vi "dfd_Render TF Polynomial.vi"(4 "alignment(left, top)":T2={"horizontal"=enum."left", "vertical"=enum."bottom"}, 5 "format string":string="%.0f", 6 "rendering options":T1, 7 "Fonts Input":T3(array[cluster]), 8 "variable":string="s", 9 "origin":cluster{"x":i16, "y":i16}={"x"=60, "y"=30}, 10 "coefficients":dbl[](array[numeric]) format="%.2f", 11 "picture in":picture) -> (2 "text rect":T4={"left"=60, "top"=13, "right"=157, "bottom"=30}, 3 "rendered equation":picture)   [LabVIEW 2017, in "NI_DigFilter_Process.lvlib"]
doc: "This VI allow to render Polynomials in Picture Control in ascending/descending order of coefficients, ascending/descending order of polynomial and with negative coefficients."
uses:
  <vilib>/addons/Digital Filter Design/NI_DigFilter_Process.lvlib
panel:
  in  "Fonts Defaut":T3(array[cluster])=[{"Font Name:"="Tahoma", "Size"=13, "Strikeout?"=FALSE, "Italic?"=FALSE, "Underline?"=FALSE, "Outline?"=FALSE, "Shadow?"=FALSE, "Bold?"=FALSE}, {"Font Name:"="Tahoma", "Size"=13, "Strikeout?"=FALSE, "Italic?"=FALSE, "Underline?"=FALSE, "Outline?"=FALSE, "Shadow?"=FALSE, "Bold?"=FALSE}, {"Font Name:"="Tahoma", "Size"=11, "Strikeout?"=FALSE, "Italic?"=FALSE, "Underline?"=FALSE, "Outline?"=FALSE, "Shadow?"=FALSE, "Bold?"=FALSE}]
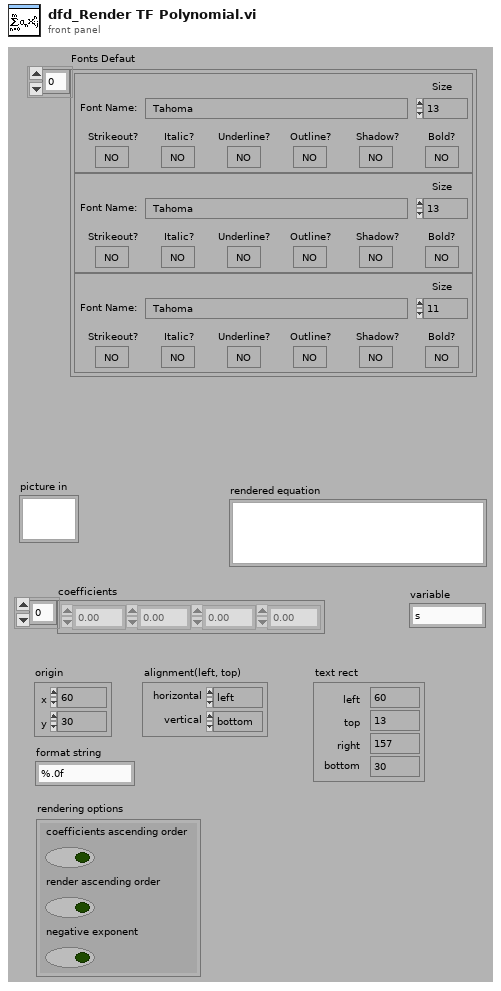
[diagram p1: front panel]
types:
  T1 = cluster{"coefficients ascending order":bool, "render ascending order":bool, "negative exponent":bool}
  T2 = cluster{"horizontal":enum16{"left", "center", "right"}, "vertical":enum16{"top", "center", "bottom"}}
  T3 = cluster{"Font Name:":string, "Size":i16, "Strikeout?":bool, "Italic?":bool, "Underline?":bool, "Outline?":bool, "Shadow?":bool, "Bold?":bool}[]
  T4 = cluster{"left":i16, "top":i16, "right":i16, "bottom":i16}
  T5 = enum16{"User-specified Font", "Application Font", "System Font", "Dialog Font"}
  T6 = cluster{"Font Name:":string, "Size":i16, "Strikeout?":bool, "Italic?":bool, "Underline?":bool, "Outline?":bool, "Shadow?":bool, "Bold?":bool}
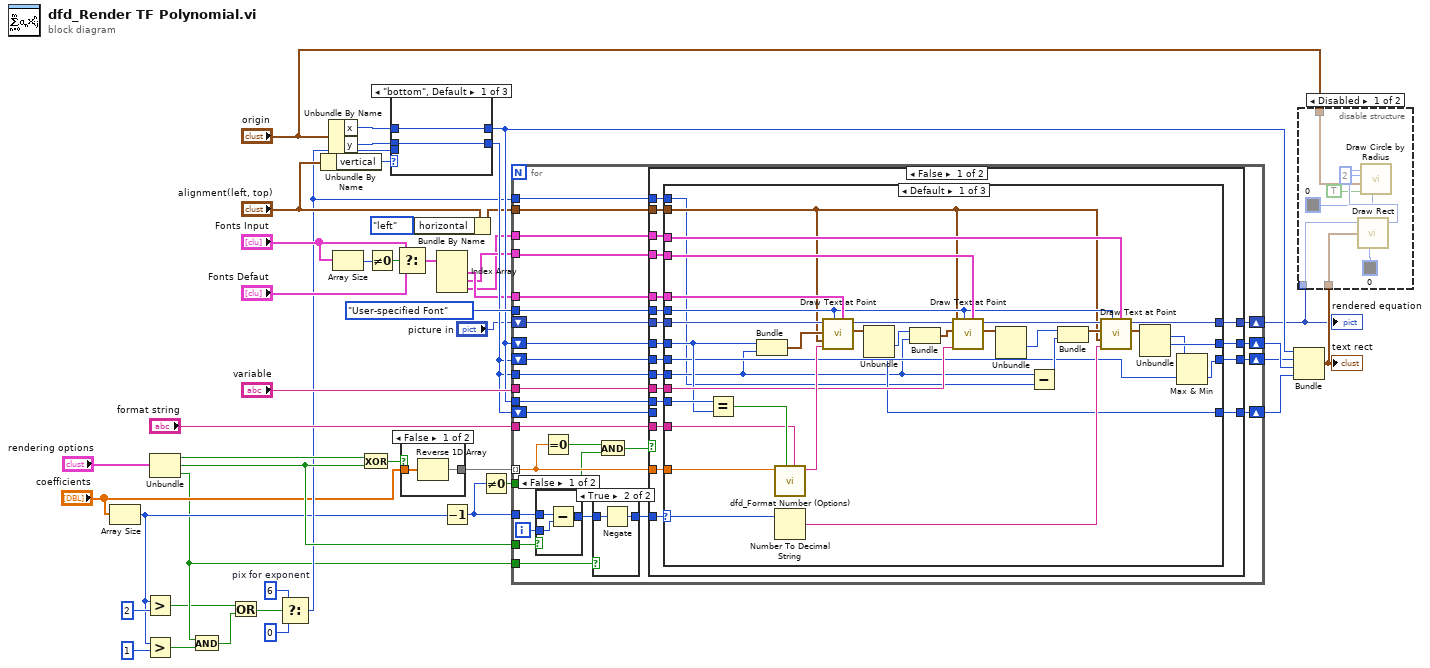
[diagram p0: block diagram]
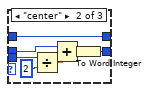
[diagram p3: hidden frame]
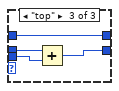
[diagram p4: hidden frame]
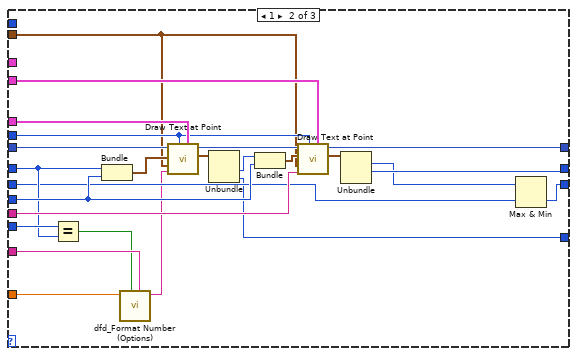
[diagram p8: hidden frame]
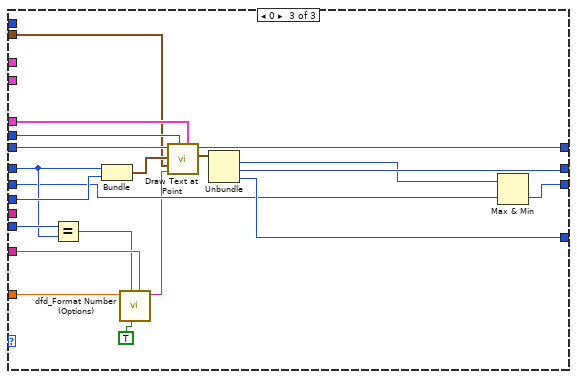
[diagram p9: hidden frame]
diagram:
  w14 = i16 6  # pix for exponent
  n1 = Array Size(array="coefficients") -> (size(s)=w4:i32)
  n2 = Greater?(x=w4, y=2) -> (0:w1:bool)
  n3 = Greater?(x=w4, y=1) -> (0:w5:bool)
  n4 = Unbundle("rendering options") -> ("coefficients ascending order"=w18:bool, "render ascending order"=w17:bool, "negative exponent"=w3:bool)
  n5 = And(x=w3, y=w5) -> (x .and. y?=w2:bool)
  n6 = Or(x=w1, y=w2) -> (x .or. y?=w7:bool)
  n7 = Select(t=w14, s=w7, f=i16 0) -> (s? t:f=w12:i16)
  n8 = Unbundle By Name("alignment(left, top)") -> ("vertical"=w15:enum16{"top", "center", "bottom"})
  n9 = Unbundle By Name("origin") -> ("x"=w26:i16, "y"=w25:i16)
  n10 = Array Size(array="Fonts Input") -> (size(s)=w36:i32)
  n11 = Exclusive Or(1:w17, 2:w18) -> (0:w28:bool)
  n12 = Not Equal To 0?(x=w36) -> (x != 0?=w37:bool)
  n13 = case shown="\"bottom\", Default" w15 {
    tunnel: [w47 w54 w58] -> w41
    tunnel: [w46 w48 w56] -> w38
    tunnel: w26 -> [w47 w54 w58]
    tunnel: w25 -> [w46 w53 w57]
    tunnel: w12 -> [_ w51 w55]
    frame "bottom", Default {
    }
    frame "center" {
      n14 = Divide(x=w51, y=i16 2) -> (x/y=w49:dbl)
      n15 = Add(x=w53, y=w49) -> (x+y=w52:dbl)
      n16 = To Word Integer(number=w52) -> (16bit integer=w48:i16)
    }
    frame "top" {
      n17 = Add(x=w57, y=w55) -> (x+y=w56:i16)
    }
  }
  n18 = Select(t="Fonts Input", s=w37, f="Fonts Defaut") -> (s? t:f=w34:T3)
  n19 = case shown="False" w28 {
    tunnel: "coefficients" -> [w60 w61]
    tunnel: [w59 w61] -> w39
    frame False {
      n20 = Reverse 1D Array(array=w60) -> (reversed array=w59:dbl[])
    }
    frame True {
    }
  }
  n21 = Bundle By Name(cluster="alignment(left, top)", "horizontal"=enum16{"left", "center", "right"}."left") -> (w23:T2)
  n22 = Index Array(array=w34) -> (element #1=w32:T6, element #2=w31:T6, element #3=w30:T6)  [unwired: 3 in]
  n23 = Decrement(x=w4) -> (x-1=w9:i32)
  n24 = Not Equal To 0?(x=w9) -> (x != 0?=w8:bool)
  n25 = for {
    tunnel: w39 -> [w70] mode=indexing
    shift-right: [w87] -> w11
    shift-left: "picture in" -> [w89]
    tunnel: "variable" -> [w88]
    shift-right: [w85] -> w44
    shift-left: w41 -> [w86]
    tunnel: w38 -> [w84]
    tunnel: w32 -> [w83]
    tunnel: w30 -> [w82]
    tunnel: w31 -> [w81]
    tunnel: w41 -> [w80]
    tunnel: w9 -> [w78]
    shift-right: [w76] -> w43
    shift-left: w38 -> [w77]
    tunnel: T5."User-specified Font" ("desired font(Application)") -> [w75]
    shift-right: [w74] -> w40
    shift-left: w38 -> [w73]
    tunnel: "format string" -> [w72]
    tunnel: w23 -> [w71]
    tunnel: w17 -> [w69]
    tunnel: w3 -> [w66]
    tunnel: w12 -> [w65]
    tunnel: w8 -> [w63]
    i -> [w79]
    n26 = case shown="False" w69 {
      tunnel: w79 -> [w95 w96]
      tunnel: w78 -> [w94 _]
      tunnel: [w93 w96] -> w68
      frame False {
        n27 = Subtract(x=w94, y=w95) -> (x-y=w93:i32)
      }
      frame True {
      }
    }
    n28 = Equal To 0?(x=w70) -> (x = 0?=w64:bool)
    n29 = case shown="True" w66 {
      tunnel: [w90 w91] -> w67
      tunnel: w68 -> [w90 w92]
      frame False {
      }
      frame True {
        n30 = Negate(x=w92) -> (-x=w91:i32)
      }
    }
    n31 = And(x=w64, y=w63) -> (x .and. y?=w62:bool)
    n32 = case shown="False" w62 {
      tunnel: w89 -> [w115 w198]
      tunnel: w88 -> [w114 _]
      tunnel: [w113 w198] -> w87
      tunnel: w86 -> [w112 w197]
      tunnel: [w111 w197] -> w85
      tunnel: w70 -> [w110 _]
      tunnel: w84 -> [w109 _]
      tunnel: w83 -> [w108 _]
      tunnel: w82 -> [w107 _]
      tunnel: w81 -> [w106 _]
      tunnel: w80 -> [w105 _]
      tunnel: w67 -> [w104 _]
      tunnel: w77 -> [w103 w196]
      tunnel: [w102 w196] -> w76
      tunnel: w75 -> [w101 _]
      tunnel: [w100 w195] -> w74
      tunnel: w73 -> [_ w195]
      tunnel: w72 -> [w99 _]
      tunnel: w71 -> [w98 _]
      tunnel: w65 -> [w97 _]
      frame False {
        n33 = case shown="Default" w104 {
          selector: w104 -> [w117 _ _]
          tunnel: w115 -> [w149 w174 w194]
          tunnel: w114 -> [w131 w164 _]
          tunnel: [w144 w161 w186] -> w113
          tunnel: w112 -> [w129 w162 w188]
          tunnel: [w127 w160 w187] -> w111
          tunnel: w110 -> [w119 w151 w177]
          tunnel: w109 -> [w118 w168 w190]
          tunnel: w108 -> [w140 w171 w191]
          tunnel: w107 -> [w141 _ _]
          tunnel: w106 -> [w134 w166 _]
          tunnel: w105 -> [w130 w163 w189]
          tunnel: w103 -> [w126 w159 w182]
          tunnel: [w124 w158 w180] -> w102
          tunnel: w101 -> [w123 w157 w185]
          tunnel: [w122 w156 w184] -> w100
          tunnel: w99 -> [w121 w153 w179]
          tunnel: w98 -> [w120 w155 w183]
          tunnel: w97 -> [w116 _ _]
          frame Default {
            n34 = Equal?(x=w130, y=w129) -> (x = y?=w128:bool)
            n35 = Bundle("x"=w129, "y"=w118) -> (w146:cluster{"x":i16, "y":i16})  [unwired: 1 out]
            n36 = call <vilib>:"dfd_Format Number (Options).vi"("format string"=w121, "Is Higher Coeffiecient?"=w128, "Coefficient"=w119) -> ("String Coefficient"=w148:string)  [unwired: 1 in, 7 out]
            n37 = Number To Decimal String(number=w117) -> (decimal integer string=w143:string)  [unwired: 1 out]
            n38 = call <vilib>:"Draw Text at Point.vi"("[user-specified font]"=w140, "desired font(Application)"=w123, "text"=w148, "alignment(left, top)"=w120, "origin"=w146, "picture"=w149) -> ("text rect"=w147:T4, "new picture"=w138:picture)  [unwired: 3 in, 1 out]
            n39 = Unbundle(w147) -> ("right"=w133:i16, "bottom"=w122:i16)  [unwired: 2 out]
            n40 = Bundle("right"=w133, "y"=w118) -> (w139:cluster{"right":i16, "y":i16})  [unwired: 1 out]
            n41 = call <vilib>:"Draw Text at Point.vi"("[user-specified font]"=w134, "desired font(Application)"=w123, "text"=w131, "alignment(left, top)"=w120, "origin"=w139, "picture"=w138) -> ("text rect"=w136:T4, "new picture"=w137:picture)  [unwired: 3 in, 1 out]
            n42 = Unbundle(w136) -> ("right"=w132:i16)  [unwired: 3 out]
            n43 = Subtract(x=w118, y=w116) -> (x-y=w142:i16)
            n44 = Bundle("right"=w132, w142) -> (w145:cluster{"right":i16, i16})  [unwired: 1 out]
            n45 = call <vilib>:"Draw Text at Point.vi"("[user-specified font]"=w141, "desired font(Application)"=w123, "text"=w143, "alignment(left, top)"=w120, "origin"=w145, "picture"=w137) -> ("text rect"=w135:T4, "new picture"=w144:picture)  [unwired: 3 in, 1 out]
            n46 = Unbundle(w135) -> ("top"=w125:i16, "right"=w127:i16)  [unwired: 2 out]
            n47 = Max & Min(x=w125, y=w126) -> (min(x,y)=w124:i16)  [unwired: 1 out]
          }
          frame 1 {
            n48 = Equal?(x=w163, y=w162) -> (x = y?=w152:bool)
            n49 = Bundle("x"=w162, "y"=w168) -> (w172:cluster{"x":i16, "y":i16})  [unwired: 1 out]
            n50 = call <vilib>:"dfd_Format Number (Options).vi"("format string"=w153, "Is Higher Coeffiecient?"=w152, "Coefficient"=w151) -> ("String Coefficient"=w150:string)  [unwired: 1 in, 7 out]
            n51 = call <vilib>:"Draw Text at Point.vi"("[user-specified font]"=w171, "desired font(Application)"=w157, "text"=w150, "alignment(left, top)"=w155, "origin"=w172, "picture"=w174) -> ("text rect"=w173:T4, "new picture"=w169:picture)  [unwired: 3 in, 1 out]
            n52 = Unbundle(w173) -> ("right"=w165:i16, "bottom"=w156:i16)  [unwired: 2 out]
            n53 = Bundle("right"=w165, "y"=w168) -> (w170:cluster{"right":i16, "y":i16})  [unwired: 1 out]
            n54 = call <vilib>:"Draw Text at Point.vi"("[user-specified font]"=w166, "desired font(Application)"=w157, "text"=w164, "alignment(left, top)"=w155, "origin"=w170, "picture"=w169) -> ("text rect"=w167:T4, "new picture"=w161:picture)  [unwired: 3 in, 1 out]
            n55 = Unbundle(w167) -> ("top"=w154:i16, "right"=w160:i16)  [unwired: 2 out]
            n56 = Max & Min(x=w154, y=w159) -> (min(x,y)=w158:i16)  [unwired: 1 out]
          }
          frame 0 {
            n57 = Equal?(x=w189, y=w188) -> (x = y?=w178:bool)
            n58 = Bundle("x"=w188, "y"=w190) -> (w192:cluster{"x":i16, "y":i16})  [unwired: 1 out]
            n59 = call <vilib>:"dfd_Format Number (Options).vi"("format string"=w179, "Is Lower Coefficient?"=TRUE ("Is Lower Coeffiecient? 2"), "Is Higher Coeffiecient?"=w178, "Coefficient"=w177) -> ("String Coefficient"=w176:string)  [unwired: 7 out]
            n60 = call <vilib>:"Draw Text at Point.vi"("[user-specified font]"=w191, "desired font(Application)"=w185, "text"=w176, "alignment(left, top)"=w183, "origin"=w192, "picture"=w194) -> ("text rect"=w193:T4, "new picture"=w186:picture)  [unwired: 3 in, 1 out]
            n61 = Unbundle(w193) -> ("top"=w181:i16, "right"=w187:i16, "bottom"=w184:i16)  [unwired: 1 out]
            n62 = Max & Min(x=w181, y=w182) -> (min(x,y)=w180:i16)  [unwired: 1 out]
          }
        }
      }
      frame True {
      }
    }
  }
  "rendered equation" <- w11
  n63 = Bundle("x"=w41, "y"=w43, "x"=w44, "y"=w40) -> (w27:cluster{"x":i16, "y":i16, "x":i16, "y":i16})  [unwired: 1 out]
  "text rect" <- w27
  n64 = disable-structure shown="Disabled" {
    disable-tunnel: w27 -> [w201 _]
    disable-tunnel: "origin" -> [w200 _]
    disable-tunnel: w11 -> [w199 _]
    frame Disabled {
      n65 = call <vilib>:"Draw Rect.vi"("picture"=w199, "rect"=w201, "color(black)"=u32 0) -> ("new picture"=w206:picture)  [unwired: 6 in]
      n66 = call <vilib>:"Draw Circle by Radius.vi"("color(black)"=u32 0, "fill?(F)"=TRUE, "pixel center"=w200, "radius"=i16 2, "picture"=w206) -> ()  [unwired: 6 in, 1 out]
    }
    frame Enabled {
    }
  }
